vi "FPGAmain_5782_Input_only.vi"() -> ()   [LabVIEW 2013]
uses:
  FPGA/DataMode.ctl
  FPGA/Input_5782/5782_states.ctl
  <vilib>/Platform/TimedLoop/XDataNode/timing_clust.ctl
  <vilib>/Platform/TimedLoop/XDataNode/nitl_modes.ctl
  <vilib>/Platform/TimedLoop/XDataNode/wakeup.ctl
  <vilib>/rvi/Emulation/niFpgaSctlEmulationGetInTimedLoop.vi
  <vilib>/rvi/Emulation/niFpgaEmulationReportErrorSimple.vi
  <vilib>/rvi/Emulation/niFpgaGetClockAttributes.vi
  <vilib>/rvi/eio/common/nirviEmuTemplateMethod_errors.vi
  <vilib>/rvi/Emulation/niFpgaCriticalErrorInLSC.vi
  <vilib>/rvi/DataTransferAndStorage/Register/Emulation/niFpgaRegisterEmulationFpgaImpl.vi
  <instcachedir>/0/niFpgaRegisterEmulationFpgaImpl_DCF4BC0110594B98B44A971D60CEEC4D.lvgen/niFpgaRegisterEmulationFpgaImpl_DCF4BC0110594B98B44A971D60CEEC4D_015.vi
  <vilib>/rvi/DataTransferAndStorage/Container/Common/niFpgaContainerGetUniqueNameForEmu.vi
  <vilib>/rvi/FIFO/Fifo_Resource/nirvififoEmulationReadFpgaImpl.vi
  <vilib>/rvi/interface/RandomDataEmulation/nirviRandomDataMultiElementFPGAFIFO.vi
  <instcachedir>/0/nirviRandomDataMultiElementFPGAFIFO_F2B80EDE0D7944A08478D8D26097D4DB.lvgen/nirviRandomDataMultiElementFPGAFIFO_F2B80EDE0D7944A08478D8D26097D4DB_005.vi
  <vilib>/rvi/interface/RandomDataEmulation/niFpgaRandomDataHandleErrors.vi
  <instcachedir>/0/niFpgaRegisterEmulationFpgaImpl_DCF4BC0110594B98B44A971D60CEEC4D.lvgen/niFpgaRegisterEmulationFpgaImpl_DCF4BC0110594B98B44A971D60CEEC4D_009.vi
  <vilib>/rvi/interface/RandomDataEmulation/nirviRandomDataFPGAFIFO.vi
  <instcachedir>/0/niFpgaRegisterEmulationFpgaImpl_DCF4BC0110594B98B44A971D60CEEC4D.lvgen/niFpgaRegisterEmulationFpgaImpl_DCF4BC0110594B98B44A971D60CEEC4D_005.vi
  <vilib>/rvi/FIFO/Fifo_Resource/nirvififoEmulationWriteFpgaImpl.vi
  <vilib>/Platform/TimedLoop/XDataNode/XDataNode.xnode
  <vilib>/eio/EIONode/EIONode.xnode
  <vilib>/rvi/DataTransferAndStorage/Container/XNode/niFpgaContainer.xnode
  <vilib>/rvi/DataTransferAndStorage/Register/Emulation/niFpgaRegisterEmulation.vi
  <vilib>/rvi/FIFO/Fifo_Resource/nirvififoEmulationRead.vi
  <vilib>/rvi/interface/RandomDataEmulation/nirviRandomDataFpgaMultiElementTemplate.vi
  <vilib>/rvi/interface/RandomDataEmulation/nirviRandomDataFpgaReadWriteTemplate.vi
  <vilib>/rvi/FIFO/Fifo_Resource/nirvififoEmulationWrite.vi
  <vilib>/Platform/TimedLoop/XDataNode/XDNodeRunTimeDep.lvlib
  <instrlib>/FlexRIO/Libraries/Helper VIs/Counters/NI FlexRIO Counters.lvlib
panel:
  out "5782 triggered":bool
  out "IO loop count":u32
  out "40M loop count":u32
  out "counter":u16
  out "state":T1
  out "host loop count":u32
  in  "IO Module\\AO Data Sync":bool=TRUE
  in  "IO Module\\SPI Write Data":u16
  out "IO Module\\SPI Read Data":u8
  in  "IO Module\\SPI Read":bool
  in  "IO Module\\SPI Write":bool
  in  "IO Module\\SPI Address":u16
  in  "IO Module\\SPI Device":u8
  out "IO Module\\SPI Idle":bool
  in  "delay phase":fxp<+,64,64>
  in  "User Command Commit":bool
  in  "User Command":u8
  out "User Command Idle":bool
  out "User Command Status":u8
  in  "User Data 0":u8
  in  "User Data 1":u8
  out "PLL Locked":bool
  out "User Error":bool
  out "Configured?":bool
  in  "Continuous":bool
  in  "5782 record length":u16=4000 caption="Samples Per Trigger" min=1 step=1
  in  "Trigger Acquisition":bool
  out "IO Module\\Trigger Input":bool
  in  "Downsample":fxp<+,8,8>=1.0
  in  "new coeffs":bool
  in  "FIR coeffs":fxp<+/-,18,18>[](array[numeric])
  in  "CIC Gain":fxp<+/-,32,1>=0.00390625 format="%#_32g"
  in  "Acquisition running":bool
  in  "Simulated phase 5782":fxp<+,64,64>[](array[numeric])=[0.0, 0.0]
  in  "Mode":T2
  in  "Phase 5782":fxp<+,64,64>[](array[numeric])=[0.0, 0.0]
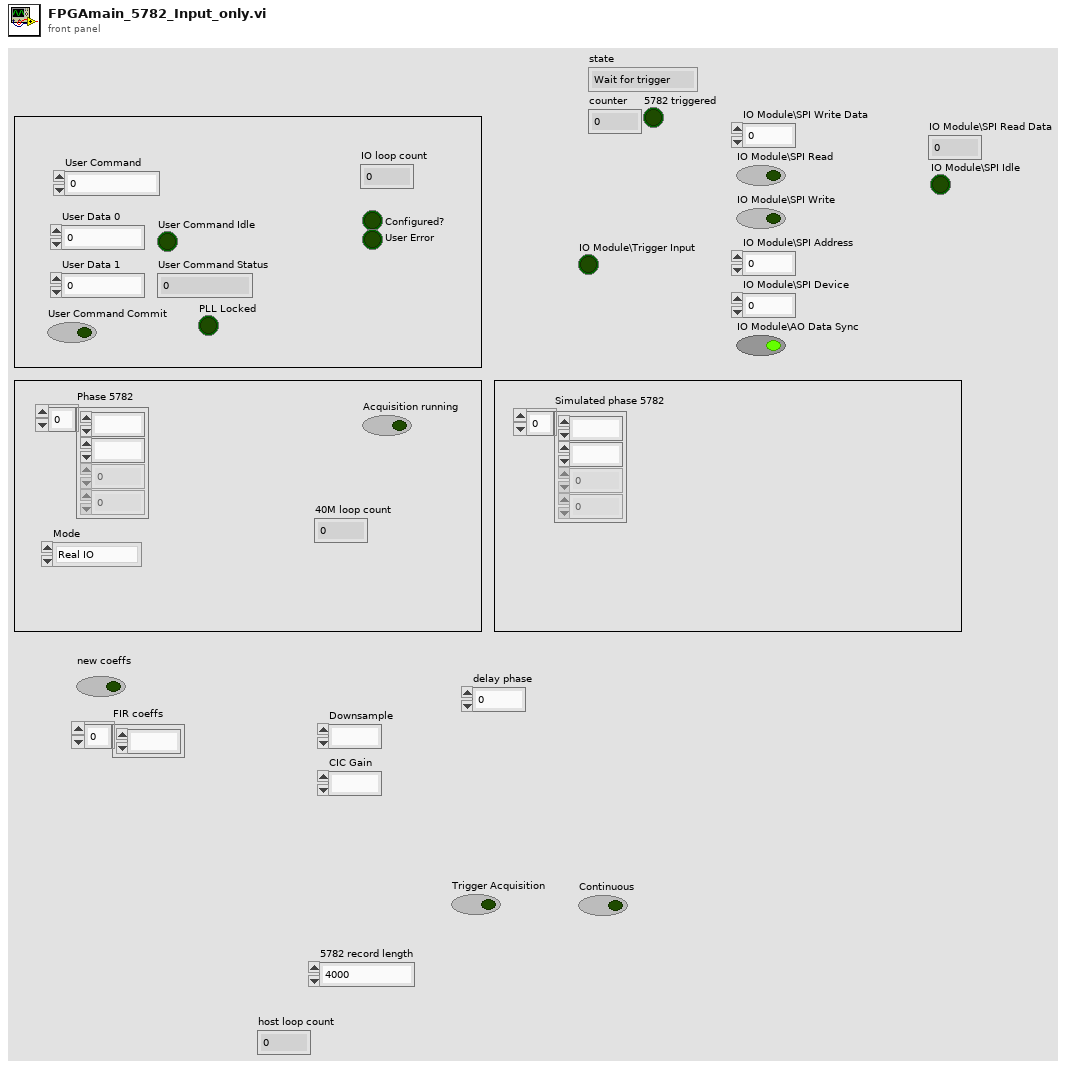
[diagram p1: front panel]
types:
  T1 = typedef "5782_states.ctl" = enum8{"Wait for trigger", "Acquisition", "Send record length", "Quiet period"}
  T2 = typedef "DataMode.ctl" = enum16{"Real IO", "Simulated"}
  T3 = typedef "XDNodeRunTimeDep.lvlib/timing_clust.ctl" = cluster{"Expected End [f-1]":u64, "Actual End [f-1]":u64, "Finished Late? [f-1]":bool, "Expected End [i-1]":u64, "Actual End [i-1]":u64, "Finished Late? [i-1]":bool, "Expected Start [i]":u64, "Actual Start [i]":u64, "Expected Start [f]":u64, "Actual Start [f]":u64, "Source Name":string, "Structure Name":string, "Period":i64, "Deadline":i64, "Offset":i64, "Start":i64, "Priority":i32, "Timeout":i32, "Mode":T4, "Wakeup Reason":T5, "Error":errorcluster, "Source Type":string, "Secondary Source Type":string, "Global End Time":u64, "Global Start Time":u64, "Frame Duration":u64, "Iteration Duration":u64, "Assigned CPU":i32, "I/O Scan Engine Mode":u32}
  T4 = typedef "XDNodeRunTimeDep.lvlib/nitl_modes.ctl" = enum32{"No Change", "Process missed periods, maintain original phase", "Discard missed periods, maintain original phase", "Process missed periods, ignore original phase", "Discard missed periods, ignore original phase"}
  T5 = typedef "XDNodeRunTimeDep.lvlib/wakeup.ctl" = enum32{"Normal", "Aborted", "Asynchronous wakeup", "Timing source error", "Timed loop error", "Timeout"}
  T6 = typedef "I16 array size 2.ctl" = i16[]
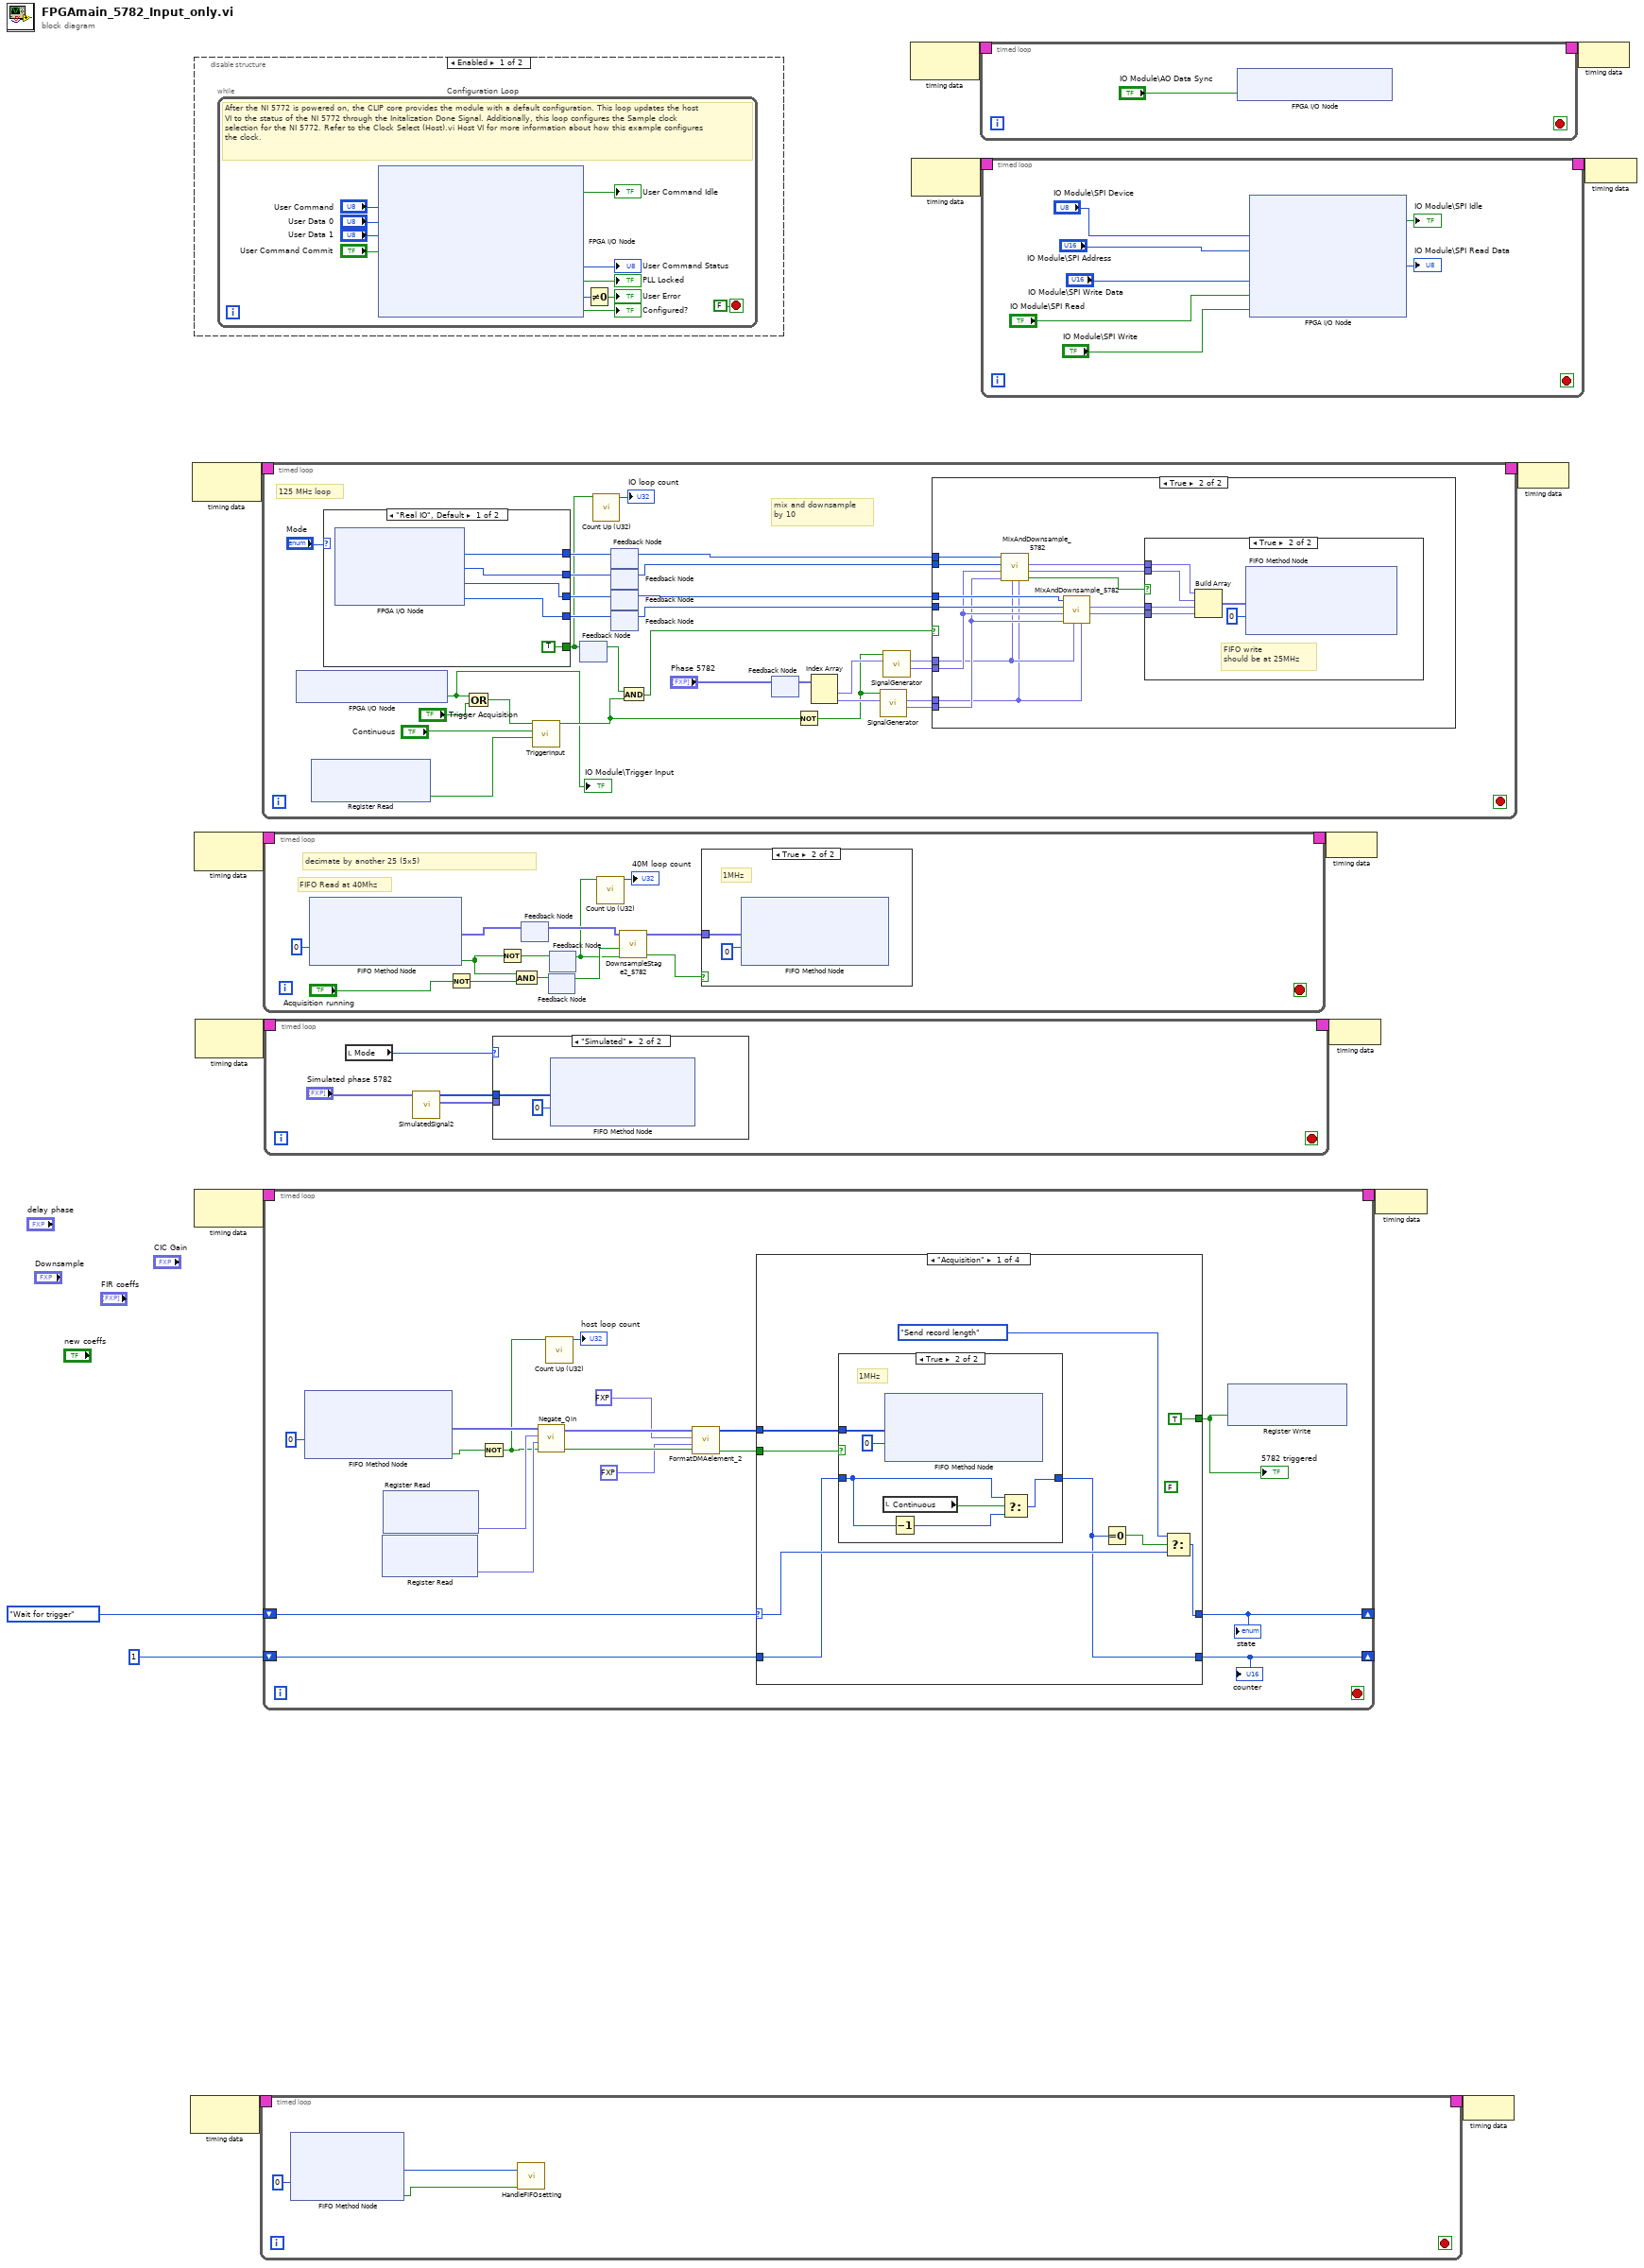
[diagram p0: block diagram]
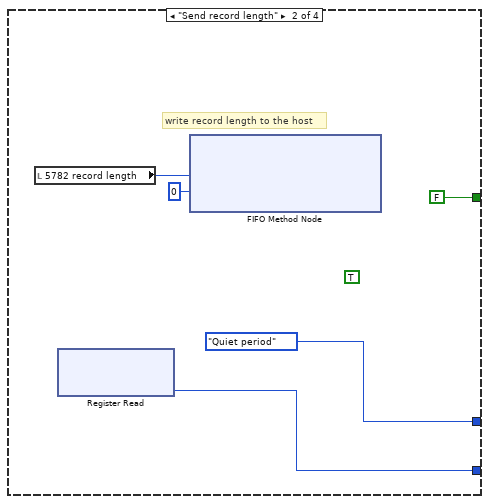
[diagram p3: hidden frame]
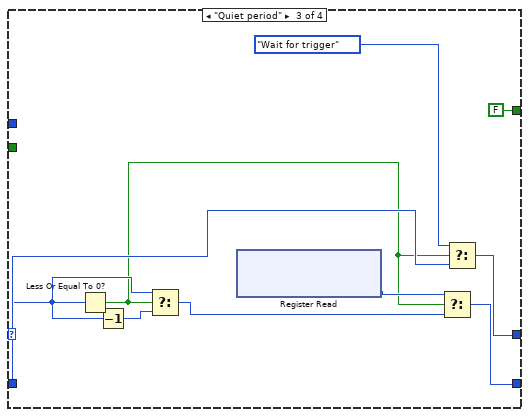
[diagram p4: hidden frame]
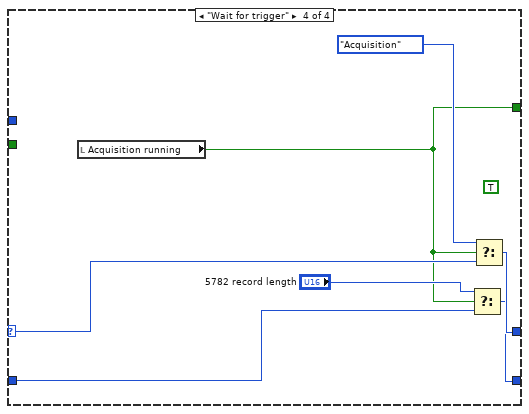
[diagram p5: hidden frame]
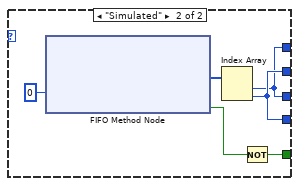
[diagram p9: hidden frame]
diagram:
  n1 = node-c288() -> (w6:T3)  [unwired: 1 in]
  n2 = node-c288() -> (w12:T3)  [unwired: 1 in]
  n3 = disable-structure shown="Enabled" {
    frame Enabled {
      n4 = while "Configuration Loop" {
        stop <- FALSE stop-if-true
        # "After the NI 5772 is powered on, the CLIP core provides the module with a default configuration. This loop updates the host VI to the status of the NI 5772 through the Initalization Done Signal. Additionally, this loop configures the Sample clock selection for the NI 5772. Refer to the Clock Select (Host).vi Host VI for more information about how this example configures the clock."
        n5 = xnode "FPGA I/O Node"("IO Module\\User Command"="User Command", "IO Module\\User Data 0"="User Data 0", "IO Module\\User Data 1"="User Data 1", "IO Module\\User Command Commit"="User Command Commit") -> ("IO Module\\User Command Idle"=→"User Command Idle":bool, "IO Module\\User Command Status"=→"User Command Status":u8, "IO Module\\PLL Locked"=→"PLL Locked":bool, "IO Module\\User Error"=w22:u8, "IO Module\\Initialization Done"=→"Configured?":bool)  [unwired: 9 in, 9 out]
        n6 = Not Equal To 0?(x=w22) -> (x != 0?=→"User Error":bool)
      }
    }
    frame Disabled {
    }
  }
  n7 = node-c288() -> (w16:T3)  [unwired: 1 in]
  n8 = node-c288() -> (w10:T3)  [unwired: 1 in]
  n9 = node-c288() -> (w14:T3)  [unwired: 1 in]
  n10 = timed-loop {
    timing: w6 -> [_]
    timing-out: [_] -> w5
    stop <- _ stop-if-true
    n11 = xnode ("FIFO Method Node")("Timeout"=0) -> ("Element"=w29:u64, "Timed Out?"=w28:bool)  [unwired: 1 in, 1 out]
    n12 = call "HandleFIFOsetting.vi"("timed out"=w28, "Value"=w29) -> ()  [unwired: 10 in]
  }
  n13 = timed-loop {
    timing: w12 -> [_]
    timing-out: [_] -> w11
    stop <- _ stop-if-true
    # "mix and downsample\nby 10"
    # "125 MHz loop"
    n14 = xnode "FPGA I/O Node"() -> ("IO Module\\Trigger Input"=w33:bool)  [unwired: 1 in, 1 out]
    "IO Module\\Trigger Input" <- w33
    n15 = xnode ("Register Read")() -> ("Data"=w36:bool)  [unwired: 1 in, 1 out]
    n16 = case shown="\"Real IO\", Default" "Mode" {
      tunnel: [w84 w87] -> w59
      tunnel: [w83 w88] -> w57
      tunnel: [w82 w87] -> w55
      tunnel: [w81 w88] -> w52
      tunnel: [TRUE w85] -> w49
      frame "Real IO", Default {
        n17 = xnode "FPGA I/O Node"() -> ("IO Module\\AI 0 N-1"=w84:i16, "IO Module\\AI 0 N"=w83:i16, "IO Module\\AI 1 N-1"=w82:i16, "IO Module\\AI 1 N"=w81:i16)  [unwired: 4 in, 4 out]
      }
      frame "Simulated" {
        n18 = xnode ("FIFO Method Node")("Timeout"=0) -> ("Element"=w89:i16[], "Timed Out?"=w86:bool)  [unwired: 1 in, 1 out]
        n19 = Index Array(array=w89) -> (element #1=w87:i16, element #2=w88:i16)  [unwired: 2 in]
        n20 = Not(x=w86) -> (.not. x?=w85:bool)
      }
    }
    n21 = Or(x=w33, y="Trigger Acquisition") -> (x .or. y?=w38:bool)
    n22 = call "TriggerInput.vi"("Ok to read"=w36, "Continous"="Continuous", "Trigger input"=w38) -> ("out"=w34:bool)  [unwired: 8 in]
    n23 = feedback #1() -> (w51:bool)  [unwired: 1 in]
    n24 = feedback-in #1(w49) -> ()
    n25 = call <instrlib>:"Count Up (U32).vi"("increment"=w49) -> ("count out"=→"IO loop count":u32)  [unwired: 14 in]
    n26 = feedback #2() -> (w58:i16)  [unwired: 1 in]
    n27 = feedback-in #2(w59) -> ()
    n28 = feedback #3() -> (w56:i16)  [unwired: 1 in]
    n29 = feedback-in #3(w57) -> ()
    n30 = feedback #4() -> (w54:i16)  [unwired: 1 in]
    n31 = feedback-in #4(w55) -> ()
    n32 = feedback #5() -> (w53:i16)  [unwired: 1 in]
    n33 = feedback-in #5(w52) -> ()
    n34 = And(x=w51, y=w34) -> (x .and. y?=w40:bool)
    n35 = feedback #6() -> (w47:fxp<+,64,64>[])  [unwired: 1 in]
    n36 = feedback-in #6("Phase 5782") -> ()
    n37 = Not(x=w34) -> (.not. x?=w39:bool)
    n38 = Index Array(array=w47) -> (element #1=w46:fxp<+,64,64>, element #2=w48:fxp<+,64,64>)  [unwired: 2 in]
    n39 = call "SignalGenerator.vi"("phase"=w48, "Reset"=w39) -> ("Cos"=w43:fxp<+/-,16,0>, "Sin"=w41:fxp<+/-,16,0>)  [unwired: 7 in, 1 out]
    n40 = call "SignalGenerator.vi"("phase"=w46, "Reset"=w39) -> ("Cos"=w44:fxp<+/-,16,0>, "Sin"=w42:fxp<+/-,16,0>)  [unwired: 7 in, 1 out]
    n41 = case shown="True" w40 {
      tunnel: w58 -> [_ w73]
      tunnel: w56 -> [_ w72]
      tunnel: w54 -> [_ w71]
      tunnel: w53 -> [_ w70]
      tunnel: w44 -> [_ w64]
      tunnel: w43 -> [_ w63]
      tunnel: w42 -> [_ w62]
      tunnel: w41 -> [_ w61]
      frame False {
      }
      frame True {
        n42 = call "MixAndDownsample_5782.vi"("sin1"=w61, "sin0"=w62, "cos1"=w63, "cos0"=w64, "signal 1"=w72, "signal 0"=w73) -> ("data valid"=w67:bool, "Q out"=w68:fxp<+/-,16,14>, "I out"=w69:fxp<+/-,16,14>)  [unwired: 3 in]
        n43 = call "MixAndDownsample_5782.vi"("sin1"=w61, "sin0"=w62, "cos1"=w63, "cos0"=w64, "signal 1"=w70, "signal 0"=w71) -> ("Q out"=w65:fxp<+/-,16,14>, "I out"=w66:fxp<+/-,16,14>)  [unwired: 3 in, 1 out]
        n44 = case shown="True" w67 {
          tunnel: w68 -> [_ w79]
          tunnel: w69 -> [_ w76]
          tunnel: w66 -> [_ w75]
          tunnel: w65 -> [_ w74]
          frame False {
          }
          frame True {
            # "FIFO write\nshould be at 25MHz"
            n45 = Build Array(w76, w79, w75, w74) -> (w78:fxp<+/-,16,14>[])
            n46 = xnode ("FIFO Method Node")("Element"=w78, "Timeout"=0) -> ()  [unwired: 1 in, 2 out]
          }
        }
      }
    }
  }
  n47 = timed-loop {
    timing: w16 -> [_]
    timing-out: [_] -> w15
    stop <- _ stop-if-true
    # "FIFO Read at 40Mhz"
    # "decimate by another 25 (5x5)"
    n48 = xnode ("FIFO Method Node")("Timeout"=0) -> ("Element"=w99:fxp<+/-,16,14>[], "Timed Out?"=w101:bool)  [unwired: 1 in, 1 out]
    n49 = Not(x="Acquisition running") -> (.not. x?=w102:bool)
    n50 = Not(x=w101) -> (.not. x?=w95:bool)
    n51 = And(x=w101, y=w102) -> (x .and. y?=w97:bool)
    n52 = feedback #7() -> (w98:fxp<+/-,16,14>[])  [unwired: 1 in]
    n53 = feedback-in #7(w99) -> ()
    n54 = feedback #8() -> (w96:bool)  [unwired: 1 in]
    n55 = feedback-in #8(w97) -> ()
    n56 = feedback #9() -> (w93:bool)  [unwired: 1 in]
    n57 = feedback-in #9(w95) -> ()
    n58 = call <instrlib>:"Count Up (U32).vi"("increment"=w93) -> ("count out"=→"40M loop count":u32)  [unwired: 14 in]
    n59 = call "DownsampleStage2_5782.vi"("valid in"=w93, "reset"=w96, "Data in"=w98) -> ("valid out"=w103:bool, "data out"=w104:fxp<+/-,16,14>[])  [unwired: 7 in]
    n60 = case shown="True" w103 {
      tunnel: w104 -> [_ w106]
      frame False {
      }
      frame True {
        # "1MHz"
        n61 = xnode ("FIFO Method Node")("Element"=w106, "Timeout"=0) -> ()  [unwired: 1 in, 2 out]
      }
    }
  }
  n62 = timed-loop {
    timing: w10 -> [_]
    timing-out: [_] -> w9
    shift-right: [w125] -> _
    shift-left: 5782_states."Wait for trigger" ("5782 states") -> [w127]
    shift-right: [w124] -> _
    shift-left: u16 1 ("trigger samples") -> [w126]
    stop <- _ stop-if-true
    n63 = xnode ("FIFO Method Node")("Timeout"=0) -> ("Element"=w116:fxp<+/-,16,14>[], "Timed Out?"=w122:bool)  [unwired: 1 in, 1 out]
    n64 = xnode ("Register Read")() -> ("Data"=w117:fxp<+/-,16,14>)  [unwired: 1 in, 1 out]
    n65 = xnode ("Register Read")() -> ("Data"=w118:fxp<+/-,16,14>)  [unwired: 1 in, 1 out]
    n66 = Not(x=w122) -> (.not. x?=w110:bool)
    n67 = call "Negate_Qin.vi"("valid in"=w110, "DC offset chan 1"=w117, "DC offset chan 0"=w118, "Data in"=w116) -> ("valid out"=w114:bool, "Data out"=w115:fxp<+/-,16,14>[])  [unwired: 6 in]
    n68 = call <instrlib>:"Count Up (U32).vi"("increment"=w110) -> ("count out"=→"host loop count":u32)  [unwired: 14 in]
    n69 = call "FormatDMAelement_2.vi"("valid in"=w114, "c(t) - AM"=fxp<+/-,32,21> 0.0, "c(t) - Phase"=fxp<+/-,32,4> 0.0, "Data in"=w115) -> ("valid out"=w120:bool, "Element"=w121:u64[])  [unwired: 6 in]
    n70 = case shown="\"Acquisition\"" w127 {
      selector: w127 -> [w136 _ w157 w165]
      tunnel: w126 -> [w132 _ w152 w159]
      tunnel: [w135 5782_states."Quiet period" ("5782 states") w156 w164] -> w125
      tunnel: [w129 w144 w158 w163] -> w124
      tunnel: w121 -> [w130 _ _ _]
      tunnel: w120 -> [w131 _ _ _]
      tunnel: [TRUE FALSE ("5782 triggered") FALSE ("5782 triggered") w160] -> w119
      frame "Acquisition" {
        (unwired) FALSE
        n71 = case shown="True" w131 {
          tunnel: w130 -> [_ w143]
          tunnel: [w137 w140] -> w129
          tunnel: w132 -> [w137 w138]
          frame False {
          }
          frame True {
            # "1MHz"
            n72 = local read "Continuous"() -> (w141:bool)
            n73 = xnode ("FIFO Method Node")("Element"=w143, "Timeout"=0) -> ()  [unwired: 1 in, 2 out]
            n74 = Decrement(x=w138) -> (x-1=w139:u16)
            n75 = Select(t=w138, s=w141, f=w139) -> (s? t:f=w140:u16)
          }
        }
        n76 = Equal To 0?(x=w129) -> (x = 0?=w133:bool)
        n77 = Select(t=5782_states."Send record length" ("5782 states"), s=w133, f=w136) -> (s? t:f=w135:T1)
      }
      frame "Send record length" {
        (unwired) TRUE
        # "write record length to the host"
        n78 = local read "5782 record length"() -> (w146:u16)
        n79 = xnode ("Register Read")() -> ("Data"=w144:u16)  [unwired: 1 in, 1 out]
        n80 = xnode ("FIFO Method Node")("Element"=w146, "Timeout"=0) -> ()  [unwired: 1 in, 2 out]
      }
      frame "Quiet period" {
        n81 = Less Or Equal To 0?(x=w152) -> (x <= 0?=w149:bool)
        n82 = Decrement(x=w152) -> (x-1=w153:u16)
        n83 = Select(t=w152, s=w149, f=w153) -> (s? t:f=w151:u16)
        n84 = xnode ("Register Read")() -> ("Data"=w150:u16)  [unwired: 1 in, 1 out]
        n85 = Select(t=w150, s=w149, f=w151) -> (s? t:f=w158:u16)
        n86 = Select(t=5782_states."Wait for trigger" ("5782 states"), s=w149, f=w157) -> (s? t:f=w156:T1)
      }
      frame "Wait for trigger" {
        (unwired) TRUE
        n87 = local read "Acquisition running"() -> (w160:bool)
        n88 = Select(t="5782 record length", s=w160, f=w159) -> (s? t:f=w163:u16)
        n89 = Select(t=5782_states."Acquisition" ("5782 states"), s=w160, f=w165) -> (s? t:f=w164:T1)
      }
    }
    "state" <- w125
    "counter" <- w124
    "5782 triggered" <- w119
    n90 = xnode ("Register Write")("Data"=w119) -> ()  [unwired: 1 in, 1 out]
  }
  n91 = timed-loop {
    timing: w14 -> [_]
    timing-out: [_] -> w13
    stop <- _ stop-if-true
    n92 = local read "Mode"() -> (w171:T2)
    n93 = call "SimulatedSignal2.vi"("Phase"="Simulated phase 5782") -> ("dummy do not use"=w168:fxp<+/-,16,0>[], "output"=w170:T6)  [unwired: 9 in]
    n94 = case shown="\"Simulated\"" w171 {
      tunnel: w170 -> [_ w172]
      tunnel: w168 -> [_ _]
      frame "Real IO", Default {
      }
      frame "Simulated" {
        n95 = xnode ("FIFO Method Node")("Element"=w172, "Timeout"=0) -> ()  [unwired: 1 in, 2 out]
      }
    }
  }
  n96 = node-c288() -> (w2:T3)  [unwired: 1 in]
  n97 = node-c288() -> (w4:T3)  [unwired: 1 in]
  n98 = timed-loop {
    timing: w2 -> [_]
    timing-out: [_] -> w1
    stop <- _ stop-if-true
    n99 = xnode "FPGA I/O Node"("IO Module\\AO Data Sync"="IO Module\\AO Data Sync") -> ()  [unwired: 1 in, 1 out]
  }
  n100 = timed-loop {
    timing: w4 -> [_]
    timing-out: [_] -> w3
    stop <- _ stop-if-true
    n101 = xnode "FPGA I/O Node"("IO Module\\SPI Device"="IO Module\\SPI Device", "IO Module\\SPI Address"="IO Module\\SPI Address", "IO Module\\SPI Write Data"="IO Module\\SPI Write Data", "IO Module\\SPI Read"="IO Module\\SPI Read", "IO Module\\SPI Write"="IO Module\\SPI Write") -> ("IO Module\\SPI Idle"=→"IO Module\\SPI Idle":bool, "IO Module\\SPI Read Data"=→"IO Module\\SPI Read Data":u8)  [unwired: 7 in, 7 out]
  }
  n102 = node-c288(w15) -> ()
  n103 = node-c288(w13) -> ()
  n104 = node-c288(w9) -> ()
  n105 = node-c288(w5) -> ()
  n106 = node-c288(w11) -> ()
  n107 = node-c288(w1) -> ()
  n108 = node-c288(w3) -> ()
